vi "queryStagePosition.vi"() -> (0 "error out":errorcluster, 3 "stagePosition":string)   [LabVIEW 2016]
uses:
  variables/applicationControl.vi
  variables/configDB.vi
  <vilib>/Instr/_visa.llb/VISA Configure Serial Port (Instr).vi
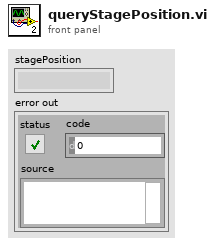
[diagram p1: front panel]
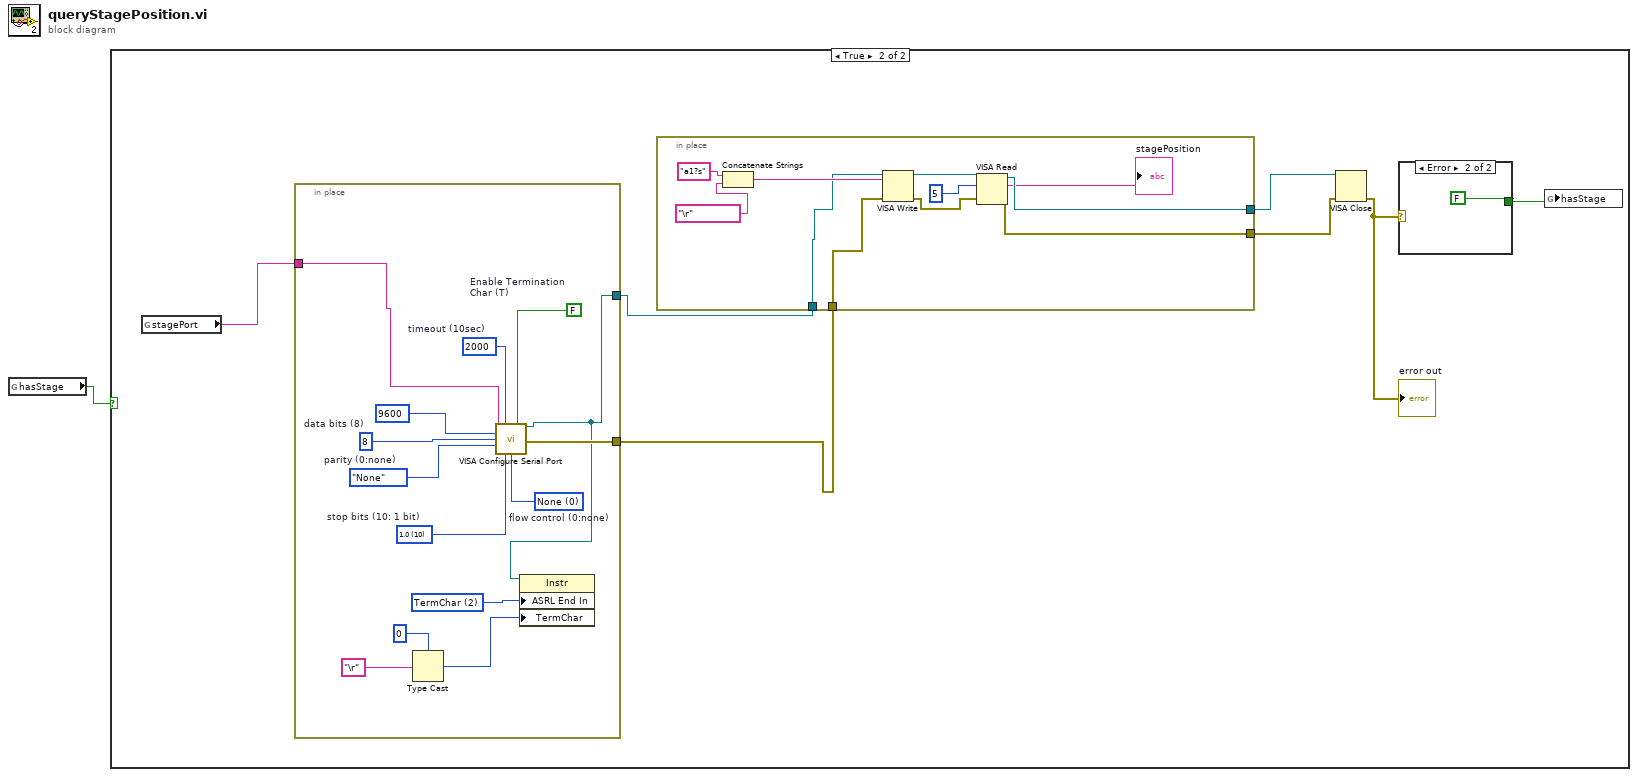
[diagram p0: block diagram]
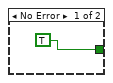
[diagram p3: hidden frame]
diagram:
  n1 = global read "applicationControl.vi" "hasStage"() -> (w1:bool)
  n2 = case shown="True" w1 {
    frame False {
    }
    frame True {
      n3 = global read "configDB.vi" "stagePort"() -> (w4:string)
      n4 = in-place {
        in-place-border: [w12] -> w8
        in-place-border: [w17] -> w7
        in-place-border: w4 -> [w11]
        w13 = u16 2 items=["None", "Last Bit", "TermChar"] ("Serial Settings:End Mode for Reads")
        w18 = u16 0 items=["None", "XON/XOFF", "RTS/CTS", "XON/XOFF & RTS/CTS", "DTR/DSR", "XON/XOFF & DTR/DSR"]  # flow control (0:none)
        w19 = u16 10 items=["1.0"=10, "1.5"=15, "2.0"=20]  # stop bits (10: 1 bit)
        w20 = FALSE  # Enable Termination Char (T)
        w21 = u32 2000  # timeout (10sec)
        w22 = enum16{"None", "Odd", "Even", "Mark", "Space"}."None"  # parity (0:none)
        w23 = u16 8  # data bits (8)
        n5 = Type Cast(type=u8 0, x="\r") -> (*(type *) &x=w15:u8)
        n6 = call-poly "VISA Configure Serial Port"("VISA resource name"=w11, "timeout (10sec)"=w21, "Enable Termination\nChar (T)"=w20, "baud rate (9600)"=u32 9600, "data bits (8)"=w23, "parity (0:none)"=w22, "stop bits (10: 1 bit)"=w19, "flow control (0:none)"=w18) -> ("VISA resource name out"=w12:refnum<visa-resource-name>, "error out"=w17:errorcluster)  [unwired: 6 in]
        n7 = property class="Instr"(reference=w12, "ASRL End In"=w13, "TermChar"=w15) -> ()  [unwired: 1 in, 2 out]
      }
      n8 = in-place {
        in-place-border: w8 -> [w30]
        in-place-border: w7 -> [w29]
        in-place-border: [w28] -> w6
        in-place-border: [w27] -> w5
        n9 = Concatenate Strings("a1?s" ("write buffer"), "\r" ("write buffer")) -> (w33:string)
        n10 = VISA Write(VISA resource name=w30, write buffer=w33, error in (no error)=w29) -> (VISA resource name out=w34:refnum<visa-resource-name>, error out=w25:errorcluster)  [unwired: 1 out]
        n11 = VISA Read(VISA resource name=w34, byte count=u32 5, error in (no error)=w25) -> (VISA resource name out=w27:refnum<visa-resource-name>, read buffer=→"stagePosition":string, error out=w28:errorcluster)  [unwired: 1 out]
      }
      n12 = VISA Close(VISA resource name=w5, error in (no error)=w6) -> (error out=w2:errorcluster)
      "error out" <- w2
      n13 = case shown="Error" w2 {
        tunnel: [TRUE FALSE] -> w3
        frame No Error {
        }
        frame Error {
        }
      }
      n14 = global write "applicationControl.vi" "hasStage"(w3) -> ()
    }
  }
